vi "multimeter_setup.vi"(8 "error in":errorcluster, 9 "Measurement":u16(ring) items=["DC Voltage (50 A - 50 mV shunt)", "DC Current (3 A terminal)", "DC Current (10 A terminal)", "AC Voltage (50 A - 50 mV shunt)", "AC Current (3 A terminal)", "AC Current (10 A terminal)", "DC Voltage (other)", "AC Voltage (other)", "Continuity", "Diode", "Frequency", "Resistance 4-wire", "Period", "Resistance 2-wire", "Temperature", "DC Voltage Ratio", "Capacitance"], 10 "Switch":bool, 11 "VISA resource name":refnum<visa-resource-name>) -> (0 "error out":errorcluster, 1 "status":bool, 2 "text":string, 3 "VISA resource name out":refnum<visa-resource-name>)   [LabVIEW 2016]
uses:
  <instrlib>/Agilent 3446X Series/Agilent 3446X Series.lvlib
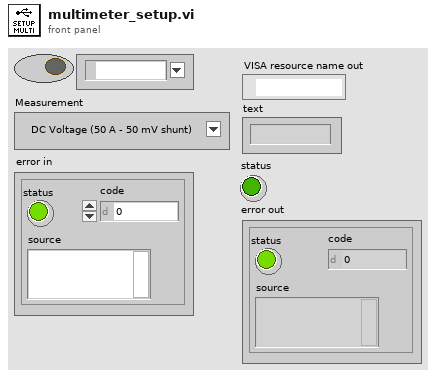
[diagram p1: front panel]
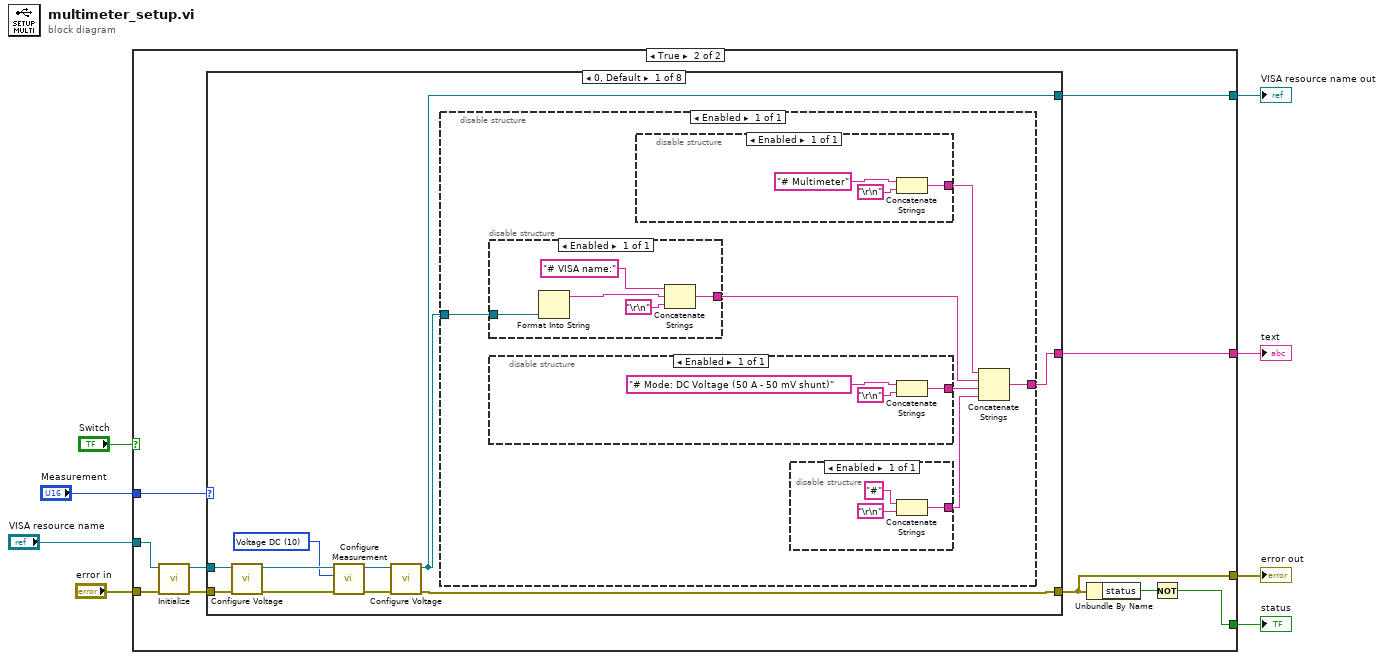
[diagram p0: block diagram]
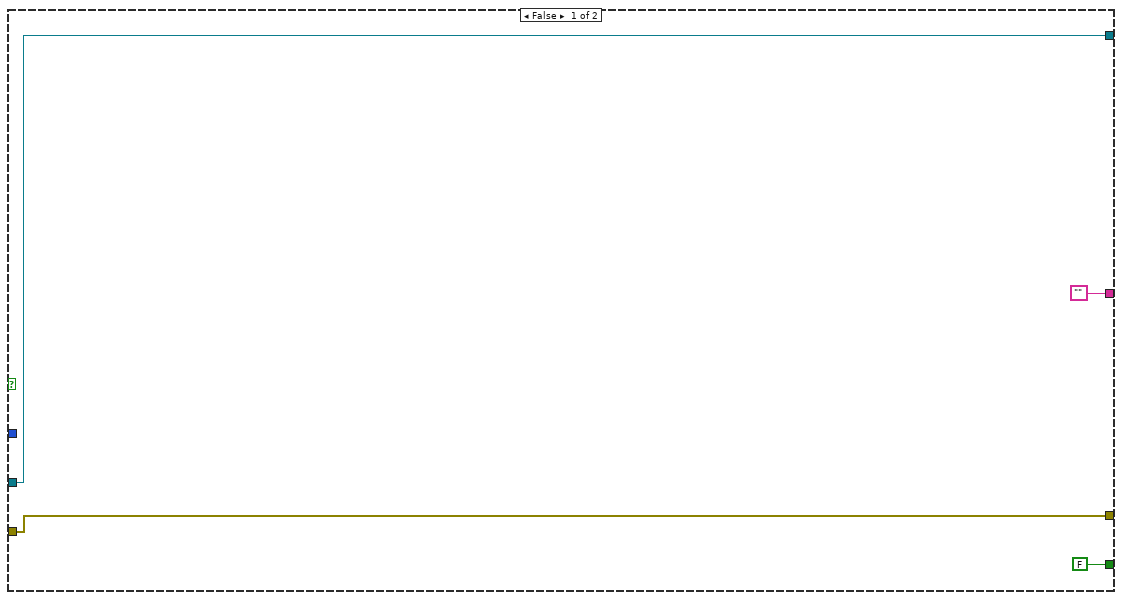
[diagram p2: hidden frame]
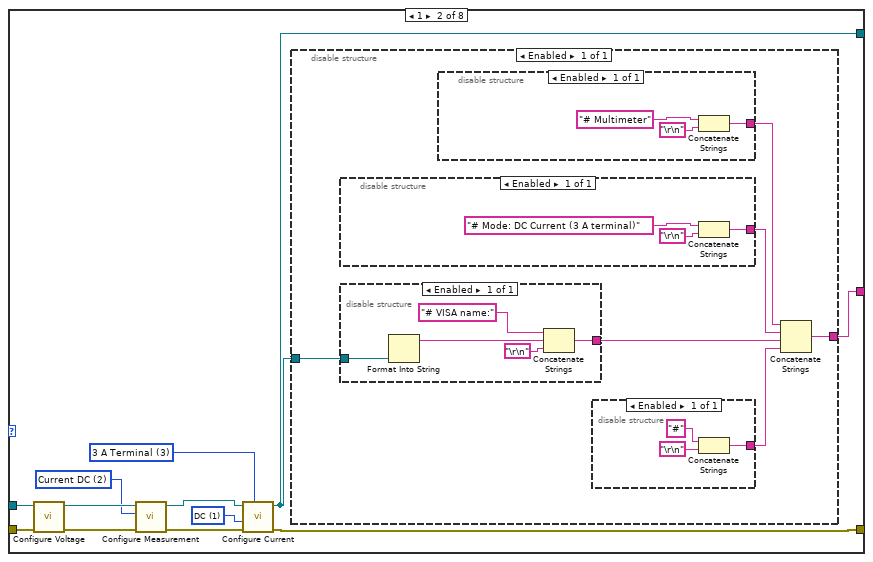
[diagram p3: hidden frame]
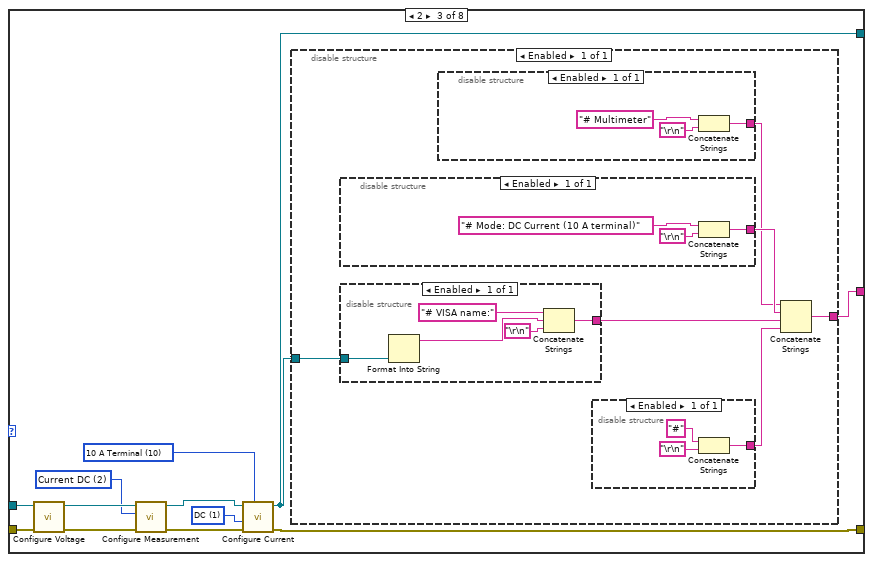
[diagram p4: hidden frame]
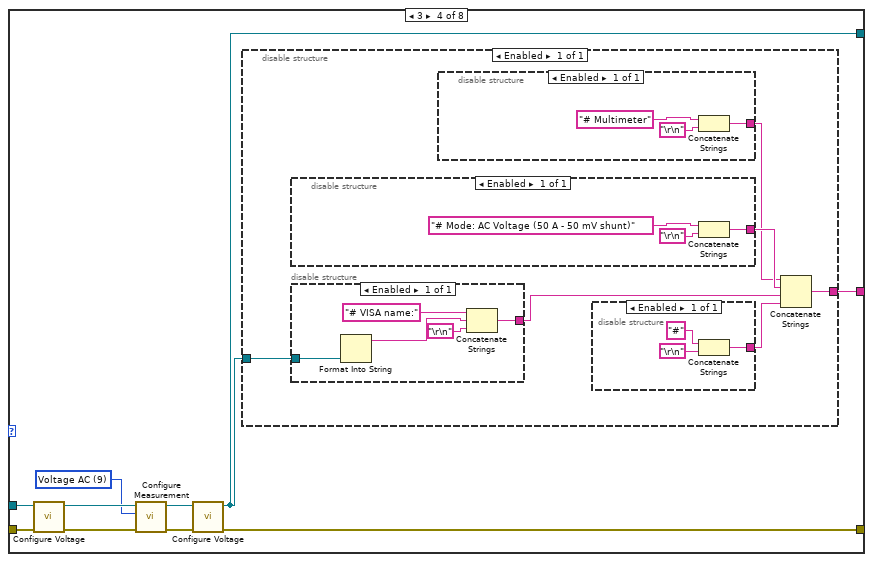
[diagram p5: hidden frame]
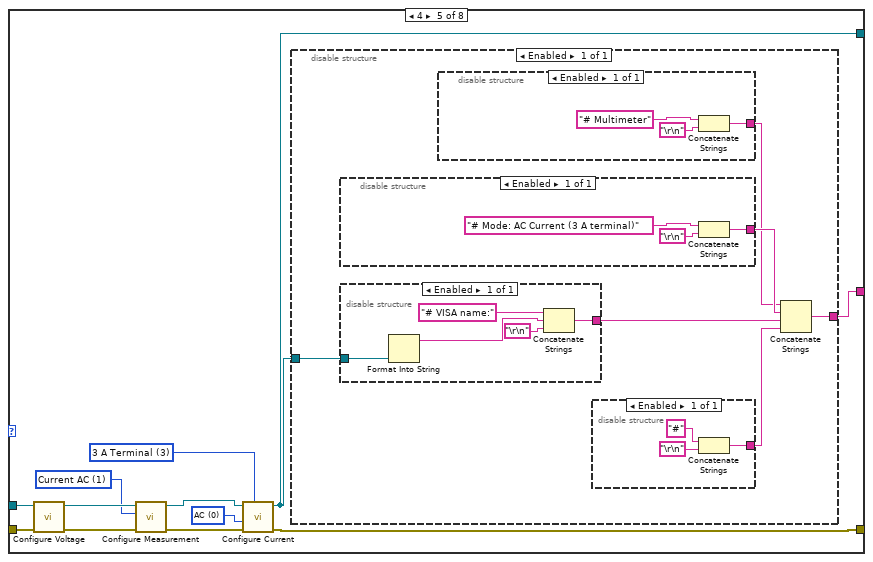
[diagram p6: hidden frame]
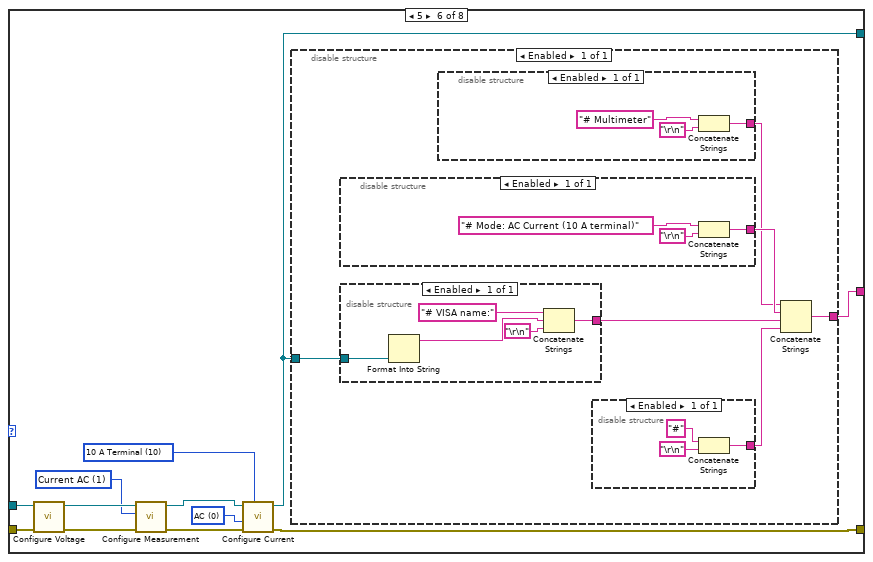
[diagram p7: hidden frame]
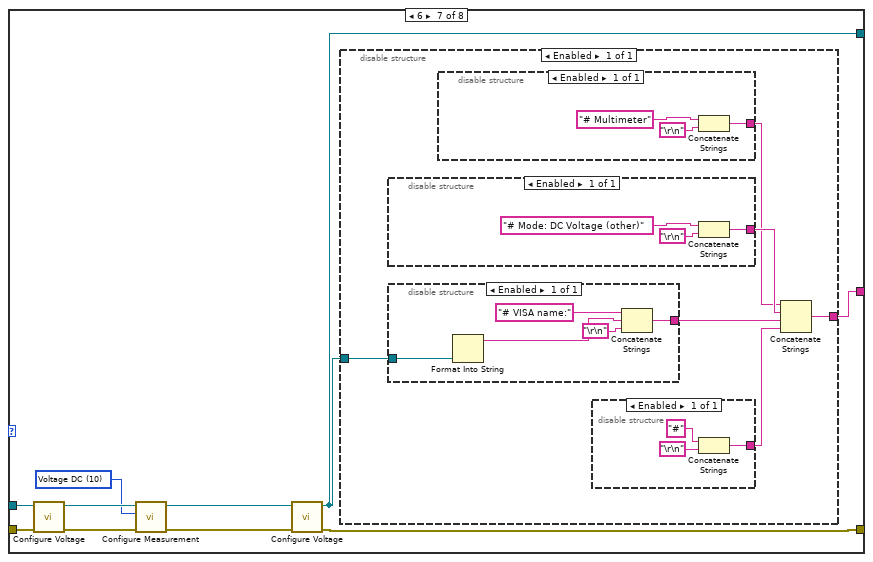
[diagram p8: hidden frame]
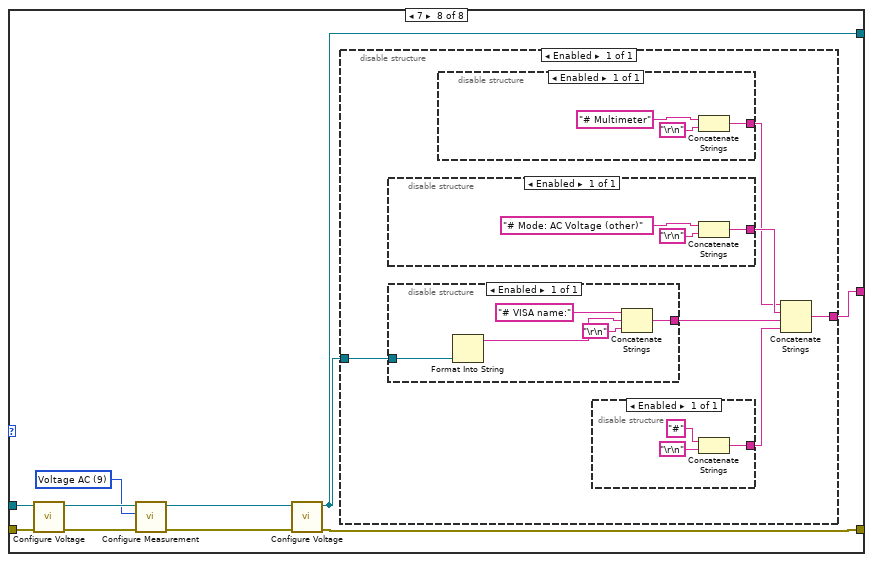
[diagram p9: hidden frame]
diagram:
  n1 = case shown="True" "Switch" {
    tunnel: [w11 w15] -> w7
    tunnel: "error in" -> [w11 w22]
    tunnel: "VISA resource name" -> [w12 w21]
    tunnel: [w12 w19] -> w3
    tunnel: "Measurement" -> [_ w17]
    tunnel: ["" w16] -> w2
    tunnel: [FALSE w14] -> w1
    frame False {
    }
    frame True {
      n2 = call <instrlib>:"Initialize.vi"("error in (no error)"=w22, "VISA resource name"=w21) -> ("error out"=w18:errorcluster, "VISA resource name out"=w20:refnum<visa-resource-name>)  [unwired: 8 in]
      n3 = case shown="0, Default" w17 {
        tunnel: [w23 w53 w85 w117 w147 w179 w211 w241] -> w19
        tunnel: w18 -> [w31 w60 w87 w118 w149 w180 w214 w242]
        tunnel: w20 -> [w32 w59 w88 w119 w150 w181 w213 w243]
        tunnel: [w25 w56 w89 w120 w148 w182 w215 w244] -> w15
        tunnel: [w24 w61 w86 w121 w151 w183 w212 w245] -> w16
        frame 0, Default {
          w28 = 10 items=["Continuity", "Current AC", "Current DC", "Diode", "Frequency", "Resistance 4-wire", "Period", "Resistance 2-wire", "Temperature", "Voltage AC", "Voltage DC", "Voltage DC Ratio", "Capacitance"] ("Measurement Function (10: Voltage DC)")
          n4 = call <instrlib>:"Configure Voltage.vi"("error in (no error)"=w31, "VISA resource name"=w32) -> ("error out"=w29:errorcluster, "VISA resource name out"=w30:refnum<visa-resource-name>)  [unwired: 8 in]
          n5 = call <instrlib>:"Configure Measurement.vi"("error in (no error)"=w29, "Measurement Function (10: Voltage DC)"=w28, "VISA resource name"=w30) -> ("error out"=w26:errorcluster, "VISA resource name out"=w27:refnum<visa-resource-name>)  [unwired: 7 in]
          n6 = call <instrlib>:"Configure Voltage.vi"("error in (no error)"=w26, "VISA resource name"=w27) -> ("error out"=w25:errorcluster, "VISA resource name out"=w23:refnum<visa-resource-name>)  [unwired: 8 in]
          n7 = disable-structure shown="Enabled" {
            disable-tunnel: [w36] -> w24
            disable-tunnel: w23 -> [w33]
            frame Enabled {
              n8 = disable-structure shown="Enabled" {
                disable-tunnel: [w42] -> w34
                disable-tunnel: w33 -> [w40]
                frame Enabled {
                  n9 = Format Into String(w40) -> (resulting string=w39:string)  [unwired: 3 in, 1 out]
                  n10 = Concatenate Strings("# VISA name:", w39, "\r\n") -> (w42:string)
                }
              }
              n11 = disable-structure shown="Enabled" {
                disable-tunnel: [w47] -> w37
                frame Enabled {
                  n12 = Concatenate Strings("# Mode: DC Voltage (50 A - 50 mV shunt)", "\r\n") -> (w47:string)
                }
              }
              n13 = disable-structure shown="Enabled" {
                disable-tunnel: [w50] -> w35
                frame Enabled {
                  n14 = Concatenate Strings("# Multimeter", "\r\n") -> (w50:string)
                }
              }
              n15 = disable-structure shown="Enabled" {
                disable-tunnel: [w44] -> w38
                frame Enabled {
                  n16 = Concatenate Strings("#", "\r\n") -> (w44:string)
                }
              }
              n17 = Concatenate Strings(w35, w34, w37, w38) -> (w36:string)
            }
          }
        }
        frame 1 {
          w54 = 3 items=["3 A Terminal"=3, "10 A Terminal"=10] ("Terminal Type (3: 3 A Terminal)")
          w55 = 1 items=["AC", "DC"] ("Current Type (0: AC)")
          w62 = 2 items=["Continuity", "Current AC", "Current DC", "Diode", "Frequency", "Resistance 4-wire", "Period", "Resistance 2-wire", "Temperature", "Voltage AC", "Voltage DC", "Voltage DC Ratio", "Capacitance"] ("Measurement Function (10: Voltage DC)")
          n18 = call <instrlib>:"Configure Voltage.vi"("error in (no error)"=w60, "VISA resource name"=w59) -> ("error out"=w63:errorcluster, "VISA resource name out"=w64:refnum<visa-resource-name>)  [unwired: 8 in]
          n19 = call <instrlib>:"Configure Measurement.vi"("error in (no error)"=w63, "Measurement Function (10: Voltage DC)"=w62, "VISA resource name"=w64) -> ("error out"=w58:errorcluster, "VISA resource name out"=w57:refnum<visa-resource-name>)  [unwired: 7 in]
          n20 = call <instrlib>:"Configure Current.vi"("Terminal Type (3: 3 A Terminal)"=w54, "error in (no error)"=w58, "Current Type (0: AC)"=w55, "VISA resource name"=w57) -> ("error out"=w56:errorcluster, "VISA resource name out"=w53:refnum<visa-resource-name>)  [unwired: 6 in]
          n21 = disable-structure shown="Enabled" {
            disable-tunnel: [w68] -> w61
            disable-tunnel: w53 -> [w65]
            frame Enabled {
              n22 = disable-structure shown="Enabled" {
                disable-tunnel: [w79] -> w70
                frame Enabled {
                  n23 = Concatenate Strings("# Mode: DC Current (3 A terminal)", "\r\n") -> (w79:string)
                }
              }
              n24 = disable-structure shown="Enabled" {
                disable-tunnel: [w74] -> w66
                disable-tunnel: w65 -> [w72]
                frame Enabled {
                  n25 = Format Into String(w72) -> (resulting string=w71:string)  [unwired: 3 in, 1 out]
                  n26 = Concatenate Strings("# VISA name:", w71, "\r\n") -> (w74:string)
                }
              }
              n27 = disable-structure shown="Enabled" {
                disable-tunnel: [w82] -> w69
                frame Enabled {
                  n28 = Concatenate Strings("# Multimeter", "\r\n") -> (w82:string)
                }
              }
              n29 = disable-structure shown="Enabled" {
                disable-tunnel: [w76] -> w67
                frame Enabled {
                  n30 = Concatenate Strings("#", "\r\n") -> (w76:string)
                }
              }
              n31 = Concatenate Strings(w69, w70, w66, w67) -> (w68:string)
            }
          }
        }
        frame 2 {
          w90 = 10 items=["3 A Terminal"=3, "10 A Terminal"=10] ("Terminal Type (3: 3 A Terminal)")
          w91 = 1 items=["AC", "DC"] ("Current Type (0: AC)")
          w94 = 2 items=["Continuity", "Current AC", "Current DC", "Diode", "Frequency", "Resistance 4-wire", "Period", "Resistance 2-wire", "Temperature", "Voltage AC", "Voltage DC", "Voltage DC Ratio", "Capacitance"] ("Measurement Function (10: Voltage DC)")
          n32 = call <instrlib>:"Configure Voltage.vi"("error in (no error)"=w87, "VISA resource name"=w88) -> ("error out"=w95:errorcluster, "VISA resource name out"=w96:refnum<visa-resource-name>)  [unwired: 8 in]
          n33 = call <instrlib>:"Configure Measurement.vi"("error in (no error)"=w95, "Measurement Function (10: Voltage DC)"=w94, "VISA resource name"=w96) -> ("error out"=w93:errorcluster, "VISA resource name out"=w92:refnum<visa-resource-name>)  [unwired: 7 in]
          n34 = call <instrlib>:"Configure Current.vi"("Terminal Type (3: 3 A Terminal)"=w90, "error in (no error)"=w93, "Current Type (0: AC)"=w91, "VISA resource name"=w92) -> ("error out"=w89:errorcluster, "VISA resource name out"=w85:refnum<visa-resource-name>)  [unwired: 6 in]
          n35 = disable-structure shown="Enabled" {
            disable-tunnel: [w100] -> w86
            disable-tunnel: w85 -> [w97]
            frame Enabled {
              n36 = disable-structure shown="Enabled" {
                disable-tunnel: [w111] -> w102
                frame Enabled {
                  n37 = Concatenate Strings("# Mode: DC Current (10 A terminal)", "\r\n") -> (w111:string)
                }
              }
              n38 = disable-structure shown="Enabled" {
                disable-tunnel: [w106] -> w98
                disable-tunnel: w97 -> [w104]
                frame Enabled {
                  n39 = Format Into String(w104) -> (resulting string=w103:string)  [unwired: 3 in, 1 out]
                  n40 = Concatenate Strings("# VISA name:", w103, "\r\n") -> (w106:string)
                }
              }
              n41 = disable-structure shown="Enabled" {
                disable-tunnel: [w114] -> w101
                frame Enabled {
                  n42 = Concatenate Strings("# Multimeter", "\r\n") -> (w114:string)
                }
              }
              n43 = disable-structure shown="Enabled" {
                disable-tunnel: [w108] -> w99
                frame Enabled {
                  n44 = Concatenate Strings("#", "\r\n") -> (w108:string)
                }
              }
              n45 = Concatenate Strings(w101, w102, w98, w99) -> (w100:string)
            }
          }
        }
        frame 3 {
          w124 = 9 items=["Continuity", "Current AC", "Current DC", "Diode", "Frequency", "Resistance 4-wire", "Period", "Resistance 2-wire", "Temperature", "Voltage AC", "Voltage DC", "Voltage DC Ratio", "Capacitance"] ("Measurement Function (10: Voltage DC)")
          n46 = call <instrlib>:"Configure Voltage.vi"("error in (no error)"=w118, "VISA resource name"=w119) -> ("error out"=w125:errorcluster, "VISA resource name out"=w126:refnum<visa-resource-name>)  [unwired: 8 in]
          n47 = call <instrlib>:"Configure Measurement.vi"("error in (no error)"=w125, "Measurement Function (10: Voltage DC)"=w124, "VISA resource name"=w126) -> ("error out"=w122:errorcluster, "VISA resource name out"=w123:refnum<visa-resource-name>)  [unwired: 7 in]
          n48 = call <instrlib>:"Configure Voltage.vi"("error in (no error)"=w122, "VISA resource name"=w123) -> ("error out"=w120:errorcluster, "VISA resource name out"=w117:refnum<visa-resource-name>)  [unwired: 8 in]
          n49 = disable-structure shown="Enabled" {
            disable-tunnel: [w130] -> w121
            disable-tunnel: w117 -> [w127]
            frame Enabled {
              n50 = disable-structure shown="Enabled" {
                disable-tunnel: [w141] -> w132
                frame Enabled {
                  n51 = Concatenate Strings("# Mode: AC Voltage (50 A - 50 mV shunt)", "\r\n") -> (w141:string)
                }
              }
              n52 = disable-structure shown="Enabled" {
                disable-tunnel: [w136] -> w129
                disable-tunnel: w127 -> [w134]
                frame Enabled {
                  n53 = Format Into String(w134) -> (resulting string=w133:string)  [unwired: 3 in, 1 out]
                  n54 = Concatenate Strings("# VISA name:", w133, "\r\n") -> (w136:string)
                }
              }
              n55 = disable-structure shown="Enabled" {
                disable-tunnel: [w144] -> w131
                frame Enabled {
                  n56 = Concatenate Strings("# Multimeter", "\r\n") -> (w144:string)
                }
              }
              n57 = disable-structure shown="Enabled" {
                disable-tunnel: [w138] -> w128
                frame Enabled {
                  n58 = Concatenate Strings("#", "\r\n") -> (w138:string)
                }
              }
              n59 = Concatenate Strings(w131, w132, w129, w128) -> (w130:string)
            }
          }
        }
        frame 4 {
          w152 = 3 items=["3 A Terminal"=3, "10 A Terminal"=10] ("Terminal Type (3: 3 A Terminal)")
          w153 = 0 items=["AC", "DC"] ("Current Type (0: AC)")
          w156 = 1 items=["Continuity", "Current AC", "Current DC", "Diode", "Frequency", "Resistance 4-wire", "Period", "Resistance 2-wire", "Temperature", "Voltage AC", "Voltage DC", "Voltage DC Ratio", "Capacitance"] ("Measurement Function (10: Voltage DC)")
          n60 = call <instrlib>:"Configure Voltage.vi"("error in (no error)"=w149, "VISA resource name"=w150) -> ("error out"=w157:errorcluster, "VISA resource name out"=w158:refnum<visa-resource-name>)  [unwired: 8 in]
          n61 = call <instrlib>:"Configure Measurement.vi"("error in (no error)"=w157, "Measurement Function (10: Voltage DC)"=w156, "VISA resource name"=w158) -> ("error out"=w155:errorcluster, "VISA resource name out"=w154:refnum<visa-resource-name>)  [unwired: 7 in]
          n62 = call <instrlib>:"Configure Current.vi"("Terminal Type (3: 3 A Terminal)"=w152, "error in (no error)"=w155, "Current Type (0: AC)"=w153, "VISA resource name"=w154) -> ("error out"=w148:errorcluster, "VISA resource name out"=w147:refnum<visa-resource-name>)  [unwired: 6 in]
          n63 = disable-structure shown="Enabled" {
            disable-tunnel: [w162] -> w151
            disable-tunnel: w147 -> [w161]
            frame Enabled {
              n64 = disable-structure shown="Enabled" {
                disable-tunnel: [w173] -> w164
                frame Enabled {
                  n65 = Concatenate Strings("# Mode: AC Current (3 A terminal)", "\r\n") -> (w173:string)
                }
              }
              n66 = disable-structure shown="Enabled" {
                disable-tunnel: [w168] -> w160
                disable-tunnel: w161 -> [w166]
                frame Enabled {
                  n67 = Format Into String(w166) -> (resulting string=w165:string)  [unwired: 3 in, 1 out]
                  n68 = Concatenate Strings("# VISA name:", w165, "\r\n") -> (w168:string)
                }
              }
              n69 = disable-structure shown="Enabled" {
                disable-tunnel: [w176] -> w163
                frame Enabled {
                  n70 = Concatenate Strings("# Multimeter", "\r\n") -> (w176:string)
                }
              }
              n71 = disable-structure shown="Enabled" {
                disable-tunnel: [w170] -> w159
                frame Enabled {
                  n72 = Concatenate Strings("#", "\r\n") -> (w170:string)
                }
              }
              n73 = Concatenate Strings(w163, w164, w160, w159) -> (w162:string)
            }
          }
        }
        frame 5 {
          w184 = 10 items=["3 A Terminal"=3, "10 A Terminal"=10] ("Terminal Type (3: 3 A Terminal)")
          w185 = 0 items=["AC", "DC"] ("Current Type (0: AC)")
          w188 = 1 items=["Continuity", "Current AC", "Current DC", "Diode", "Frequency", "Resistance 4-wire", "Period", "Resistance 2-wire", "Temperature", "Voltage AC", "Voltage DC", "Voltage DC Ratio", "Capacitance"] ("Measurement Function (10: Voltage DC)")
          n74 = call <instrlib>:"Configure Voltage.vi"("error in (no error)"=w180, "VISA resource name"=w181) -> ("error out"=w189:errorcluster, "VISA resource name out"=w190:refnum<visa-resource-name>)  [unwired: 8 in]
          n75 = call <instrlib>:"Configure Measurement.vi"("error in (no error)"=w189, "Measurement Function (10: Voltage DC)"=w188, "VISA resource name"=w190) -> ("error out"=w187:errorcluster, "VISA resource name out"=w186:refnum<visa-resource-name>)  [unwired: 7 in]
          n76 = call <instrlib>:"Configure Current.vi"("Terminal Type (3: 3 A Terminal)"=w184, "error in (no error)"=w187, "Current Type (0: AC)"=w185, "VISA resource name"=w186) -> ("error out"=w182:errorcluster, "VISA resource name out"=w179:refnum<visa-resource-name>)  [unwired: 6 in]
          n77 = disable-structure shown="Enabled" {
            disable-tunnel: [w194] -> w183
            disable-tunnel: w179 -> [w191]
            frame Enabled {
              n78 = disable-structure shown="Enabled" {
                disable-tunnel: [w205] -> w196
                frame Enabled {
                  n79 = Concatenate Strings("# Mode: AC Current (10 A terminal)", "\r\n") -> (w205:string)
                }
              }
              n80 = disable-structure shown="Enabled" {
                disable-tunnel: [w200] -> w192
                disable-tunnel: w191 -> [w198]
                frame Enabled {
                  n81 = Format Into String(w198) -> (resulting string=w197:string)  [unwired: 3 in, 1 out]
                  n82 = Concatenate Strings("# VISA name:", w197, "\r\n") -> (w200:string)
                }
              }
              n83 = disable-structure shown="Enabled" {
                disable-tunnel: [w208] -> w195
                frame Enabled {
                  n84 = Concatenate Strings("# Multimeter", "\r\n") -> (w208:string)
                }
              }
              n85 = disable-structure shown="Enabled" {
                disable-tunnel: [w202] -> w193
                frame Enabled {
                  n86 = Concatenate Strings("#", "\r\n") -> (w202:string)
                }
              }
              n87 = Concatenate Strings(w195, w196, w192, w193) -> (w194:string)
            }
          }
        }
        frame 6 {
          w218 = 10 items=["Continuity", "Current AC", "Current DC", "Diode", "Frequency", "Resistance 4-wire", "Period", "Resistance 2-wire", "Temperature", "Voltage AC", "Voltage DC", "Voltage DC Ratio", "Capacitance"] ("Measurement Function (10: Voltage DC)")
          n88 = call <instrlib>:"Configure Voltage.vi"("error in (no error)"=w214, "VISA resource name"=w213) -> ("error out"=w219:errorcluster, "VISA resource name out"=w220:refnum<visa-resource-name>)  [unwired: 8 in]
          n89 = call <instrlib>:"Configure Measurement.vi"("error in (no error)"=w219, "Measurement Function (10: Voltage DC)"=w218, "VISA resource name"=w220) -> ("error out"=w216:errorcluster, "VISA resource name out"=w217:refnum<visa-resource-name>)  [unwired: 7 in]
          n90 = call <instrlib>:"Configure Voltage.vi"("error in (no error)"=w216, "VISA resource name"=w217) -> ("error out"=w215:errorcluster, "VISA resource name out"=w211:refnum<visa-resource-name>)  [unwired: 8 in]
          n91 = disable-structure shown="Enabled" {
            disable-tunnel: [w224] -> w212
            disable-tunnel: w211 -> [w221]
            frame Enabled {
              n92 = disable-structure shown="Enabled" {
                disable-tunnel: [w235] -> w226
                frame Enabled {
                  n93 = Concatenate Strings("# Mode: DC Voltage (other)", "\r\n") -> (w235:string)
                }
              }
              n94 = disable-structure shown="Enabled" {
                disable-tunnel: [w230] -> w223
                disable-tunnel: w221 -> [w228]
                frame Enabled {
                  n95 = Format Into String(w228) -> (resulting string=w227:string)  [unwired: 3 in, 1 out]
                  n96 = Concatenate Strings("# VISA name:", w227, "\r\n") -> (w230:string)
                }
              }
              n97 = disable-structure shown="Enabled" {
                disable-tunnel: [w238] -> w225
                frame Enabled {
                  n98 = Concatenate Strings("# Multimeter", "\r\n") -> (w238:string)
                }
              }
              n99 = disable-structure shown="Enabled" {
                disable-tunnel: [w232] -> w222
                frame Enabled {
                  n100 = Concatenate Strings("#", "\r\n") -> (w232:string)
                }
              }
              n101 = Concatenate Strings(w225, w226, w223, w222) -> (w224:string)
            }
          }
        }
        frame 7 {
          w248 = 9 items=["Continuity", "Current AC", "Current DC", "Diode", "Frequency", "Resistance 4-wire", "Period", "Resistance 2-wire", "Temperature", "Voltage AC", "Voltage DC", "Voltage DC Ratio", "Capacitance"] ("Measurement Function (10: Voltage DC)")
          n102 = call <instrlib>:"Configure Voltage.vi"("error in (no error)"=w242, "VISA resource name"=w243) -> ("error out"=w249:errorcluster, "VISA resource name out"=w250:refnum<visa-resource-name>)  [unwired: 8 in]
          n103 = call <instrlib>:"Configure Measurement.vi"("error in (no error)"=w249, "Measurement Function (10: Voltage DC)"=w248, "VISA resource name"=w250) -> ("error out"=w246:errorcluster, "VISA resource name out"=w247:refnum<visa-resource-name>)  [unwired: 7 in]
          n104 = call <instrlib>:"Configure Voltage.vi"("error in (no error)"=w246, "VISA resource name"=w247) -> ("error out"=w244:errorcluster, "VISA resource name out"=w241:refnum<visa-resource-name>)  [unwired: 8 in]
          n105 = disable-structure shown="Enabled" {
            disable-tunnel: [w254] -> w245
            disable-tunnel: w241 -> [w253]
            frame Enabled {
              n106 = disable-structure shown="Enabled" {
                disable-tunnel: [w265] -> w256
                frame Enabled {
                  n107 = Concatenate Strings("# Mode: AC Voltage (other)", "\r\n") -> (w265:string)
                }
              }
              n108 = disable-structure shown="Enabled" {
                disable-tunnel: [w260] -> w251
                disable-tunnel: w253 -> [w258]
                frame Enabled {
                  n109 = Format Into String(w258) -> (resulting string=w257:string)  [unwired: 3 in, 1 out]
                  n110 = Concatenate Strings("# VISA name:", w257, "\r\n") -> (w260:string)
                }
              }
              n111 = disable-structure shown="Enabled" {
                disable-tunnel: [w268] -> w255
                frame Enabled {
                  n112 = Concatenate Strings("# Multimeter", "\r\n") -> (w268:string)
                }
              }
              n113 = disable-structure shown="Enabled" {
                disable-tunnel: [w262] -> w252
                frame Enabled {
                  n114 = Concatenate Strings("#", "\r\n") -> (w262:string)
                }
              }
              n115 = Concatenate Strings(w255, w256, w251, w252) -> (w254:string)
            }
          }
        }
      }
      n116 = Unbundle By Name(w15) -> ("status"=w13:bool)
      n117 = Not(x=w13) -> (.not. x?=w14:bool)
    }
  }
  "error out" <- w7
  "VISA resource name out" <- w3
  "text" <- w2
  "status" <- w1
